vi "IterativeImputer.vi"(8 "error in":errorcluster caption="entrée d'erreur", 11 "IterativeImputer":T1={"estimator"="None", "missing_values"="nan", "sample_posterior"=FALSE, "max_iter"=10, "tol"=0.001, "n_nearest_features"=-1, "initial_strategy"="mean", "imputation_order"="ascending", "skip_complete"=FALSE, "min_value"=["None"], "max_value"=["None"], "verbose"=0, "random_state"=-1, "add_indicator"=FALSE} {"random_state" min=-1; "n_nearest_features" min=-1}) -> (0 "error out":errorcluster caption="sortie d'erreur", 3 "IterativeImputer.lvclass":refnum<class "IterativeImputer.lvclass">)   [LabVIEW 2020]
doc: "Multivariate imputer that estimates each feature from all the others.\n\nA strategy for imputing missing values by modeling each feature with missing values as a function of other features in a round-robin fashion.\n\nParameters :\n\n- estimator : object, default=BayesianRidge()\nThe estimator to use at each step of the round-robin imputation. If sample_posterior is True, the estimator must support return_std in its predict method.\n\n- missing_values : int, np.nan, default=nan\nThe placeholder for the missing values. All occurrences of missing_values will be imputed. For pandas’ dataframes with nullable integer dtypes with missing values, missing_values should be set to np.nan, since pd.NA will be converted to np.nan.\n\n- sample_posterior : boolean, default=False\nWhether to sample from the (Gaussian) predictive posterior of the fitted estimator for each imputation. Estimator must support return_std in its predict method if set to True. Set to True if using IterativeImputer for multiple imputations.\n\n- max_iter : int, default=10\nMaximum number of imputation rounds to perform before returning the imputations computed during the final round. A round is a single imputation of each feature with missing values. The stopping criterion is met once abs(max(X_t - X_{t-1}))/abs(max(X[known_vals])) < tol, where X_t is X at iteration t. Note that early stopping is only applied if ``sample_posterior=False`.\n\n- tol : float, default=1e-3\nTolerance of the stopping condition.\n\n- n_nearest_features : int, default=None=-1\nNumber of other features to use to estimate the missing values of each feature column. Nearness between features is measured using the absolute correlation coefficient between each feature pair (after initial imputation). To ensure coverage of features throughout the imputation process, the neighbor features are not necessarily nearest, but are drawn with probability proportional to correlation for each imputed target feature. Can provide significant speed-up when the number of features is huge. If None, all features will be used.\n\n- initial_strategy : str, default=’mean’\nWhich strategy to use to initialize the missing values. Same as the strategy parameter in sklearn.impute.SimpleImputer Valid values: {“mean”, “median”, “most_frequent”, or “constant”}.\n\n- imputation_order : str, default=’ascending’\nThe order in which the features will be imputed. Possible values:\n\n“ascending”\nFrom features with fewest missing values to most.\n\n“descending”\nFrom features with most missing values to fewest.\n\n“roman”\nLeft to right.\n\n“arabic”\nRight to left.\n\n“random”\nA random order for each round.\n\n- skip_complete : boolean, default=False\nIf True then features with missing values during transform which did not have any missing values during fit will be imputed with the initial imputation method only. Set to True if you have many features with no missing values at both fit and transform time to save compute.\n\n- min_value : float or array-like of shape (n_features,), default=None.\nMinimum possible imputed value. Broadcast to shape (n_features,) if scalar. If array-like, expects shape (n_features,), one min value for each feature. None (default) is converted to -np.inf.\n\n- max_value : float or array-like of shape (n_features,), default=None.\nMaximum possible imputed value. Broadcast to shape (n_features,) if scalar. If array-like, expects shape (n_features,), one max value for each feature. None (default) is converted to np.inf.\n\n- verbose : int, default=0\nVerbosity flag, controls the debug messages that are issued as functions are evaluated. The higher, the more verbose. Can be 0, 1, or 2.\n\n- random_state : int, RandomState instance or None, default=None=-1\nThe seed of the pseudo random number generator to use. Randomizes selection of estimator features if n_nearest_features is not None, the imputation_order if random, and the sampling from posterior if sample_posterior is True. Use an integer for determinism. See the Glossary.\n\n- add_indicatorboolean, default=False\nIf True, a MissingIndicator transform will stack onto output of the imputer’s transform. This allows a predictive estimator to account for missingness despite imputation. If a feature has no missing values at fit/train time, the feature won’t appear on the missing indicator even if there are missing values at transform/test time.\n\n\n\nMethods :\n\n\n- Fit : Fits the imputer on X and return self.\n\nParameters : X : array-like, shape (n_samples, n_features)\n Input data, where “n_samples” is the number of samples and “n_features” is the number of features.\n y : ignored\n\n\n- Fit Transform : Fits the imputer on X and return the transformed X.\n\nParameters : X : array-like, shape (n_samples, n_features)\n Input data, where “n_samples” is the number of samples and “n_features” is the number of features.\n y : ignored.\n\nReturns : Xt : array-like, shape (n_samples, n_features)\n The imputed input data.\n\n\n- Transform : Imputes all missing values in X.\nNote that this is stochastic, and that if random_state is not fixed, repeated calls, or permuted input, will yield different results.\n\nParameters : X : array-like of shape (n_samples, n_features)\n The input data to complete.\n\nReturns : Xt : array-like, shape (n_samples, n_features)\n The imputed input data."
uses:
  IterativeImputer.lvclass
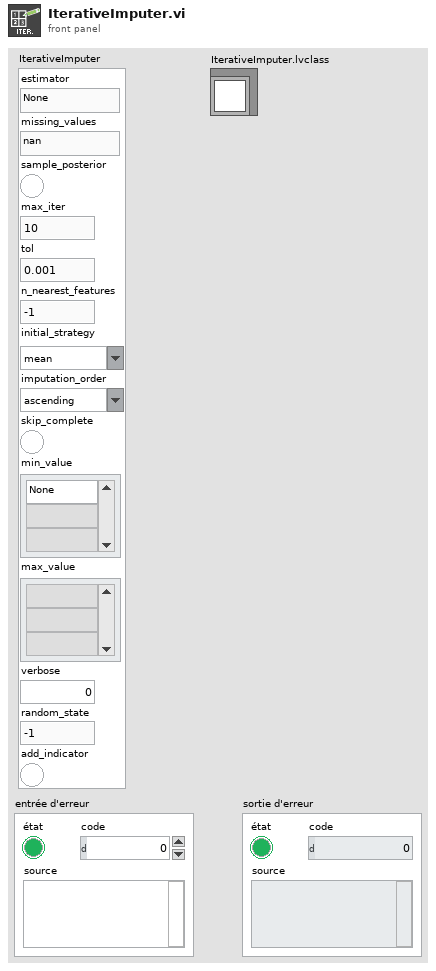
[diagram p1: front panel]
types:
  T1 = cluster{"estimator":string, "missing_values":string, "sample_posterior":bool, "max_iter":i32, "tol":dbl, "n_nearest_features":i32, "initial_strategy":string, "imputation_order":string, "skip_complete":bool, "min_value":string[], "max_value":string[], "verbose":i32, "random_state":i32, "add_indicator":bool}
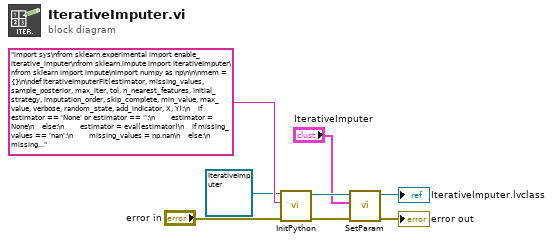
[diagram p0: block diagram]
diagram:
  n1 = call-dynamic "InitPython.vi"("error in (no error)"="error in", "Python Instruction"="import sys\nfrom sklearn.experimental import enable_iterative_imputer\nfrom sklearn.impute import IterativeImputer\nfrom sklearn import impute\nimport numpy as np\n\n\nmem = {}\n\ndef IterativeImputerFit(estimator, missing_values, sample_posterior, max_iter, tol, n_nearest_features, initial_strategy, imputation_order, skip_complete, min_value, max_value, verbose, random_state, add_indicator, X, Y):\n    if estimator == 'None' or estimator == '':\n        estimator = None\n    else:\n        estimator = eval(estimator)\n    if missing_values == 'nan':\n        missing_values = np.nan\n    else:\n        missing_values = eval(missing_values)\n    if n_nearest_features == -1:\n        n_nearest_features = None\n    if min_value == [] or min_value[0] == 'None':\n        min_value = None\n    else:\n        min_value = eval(min_value)\n    if max_value == [] or max_value[0] == 'None':\n        max_value = None\n    else:\n        max_value = eval(max_value)\n    if random_state == -1:\n        random_state = None\n    X = eval(X)\n    if Y == '':\n        Y = None\n    else:\n        Y = eval(Y)\n    try:\n        IterativeImputers = IterativeImputer(estimator, missing_values, sample_posterior, max_iter, tol, n_nearest_features, initial_strategy, imputation_order, skip_complete, min_value, max_value, verbose, random_state, add_indicator).fit(X, Y)\n        mem['FitIterativeImputer'] = IterativeImputers\n        return str('OK')\n    except:\n        erreur = sys.exc_info()\n        typerr = u\"%s\" % (erreur[0])\n        typerr = typerr[typerr.find(\"'\")+1:typerr.rfind(\"'\")]\n        msgerr = u\"%s\" % (erreur[1])\n        message = str('/!\\\\ {0} : {1}'. format(typerr,msgerr))\n        return message \n\ndef IterativeImputerFitTransform(estimator, missing_values, sample_posterior, max_iter, tol, n_nearest_features, initial_strategy, imputation_order, skip_complete, min_value, max_value, verbose, random_state, add_indicator, X, Y):\n    if estimator == 'None' or estimator == '':\n        estimator = None\n    else:\n        estimator = eval(estimator)\n    if missing_values == 'nan':\n        missing_values = np.nan\n    else:\n        missing_values = eval(missing_values)\n    if n_nearest_features == -1:\n        n_nearest_features = None\n    if min_value == [] or min_value[0] == 'None':\n        min_value = None\n    else:\n        min_value = eval(min_value)\n    if max_value == [] or max_value[0] == 'None':\n        max_value = None\n    else:\n        max_value = eval(max_value)\n    if random_state == -1:\n        random_state = None\n    X = eval(X)\n    if Y == '':\n        Y = None\n    else:\n        Y = eval(Y)\n    try:\n        IterativeImputers = IterativeImputer(estimator, missing_values, sample_posterior, max_iter, tol, n_nearest_features, initial_strategy, imputation_order, skip_complete, min_value, max_value, verbose, random_state, add_indicator).fit_transform(X, Y)\n        IterativeImputers = IterativeImputers.tolist()\n        return str(IterativeImputers)\n    except:\n        erreur = sys.exc_info()\n        typerr = u\"%s\" % (erreur[0])\n        typerr = typerr[typerr.find(\"'\")+1:typerr.rfind(\"'\")]\n        msgerr = u\"%s\" % (erreur[1])\n        message = str('/!\\\\ {0} : {1}'. format(typerr,msgerr))\n        return message \n    \n\ndef IterativeImputerTransform(estimator, missing_values, sample_posterior, max_iter, tol, n_nearest_features, initial_strategy, imputation_order, skip_complete, min_value, max_value, verbose, random_state, add_indicator, X, Y):  \n    if estimator == 'None' or estimator == '':\n        estimator = None\n    else:\n        estimator = eval(estimator)\n    if missing_values == 'nan':\n        missing_values = np.nan\n    else:\n        missing_values = eval(missing_values)\n    if n_nearest_features == -1:\n        n_nearest_features = None\n    if min_value == [] or min_value[0] == 'None':\n        min_value = None\n    else:\n        min_value = eval(min_value)\n    if max_value == [] or max_value[0] == 'None':\n        max_value = None\n    else:\n        max_value = eval(max_value)\n    if random_state == -1:\n        random_state = None\n    X = eval(X)\n    if Y == '':\n        Y = None\n    else:\n        Y = eval(Y)\n    try:\n        IterativeImputer = mem['FitIterativeImputer'].transform(X, Y)\n        IterativeImputer = IterativeImputer.tolist()\n        return str(IterativeImputer)\n    except:\n        erreur = sys.exc_info()\n        typerr = u\"%s\" % (erreur[0])\n        typerr = typerr[typerr.find(\"'\")+1:typerr.rfind(\"'\")]\n        msgerr = u\"%s\" % (erreur[1])\n        message = str('/!\\\\ {0} : {1}'. format(typerr,msgerr))\n        return message", "Scikit-learn en entrée"=refnum<class "IterativeImputer.lvclass"> refnum ("IterativeImputer.lvclass")) -> ("error out"=w6:errorcluster, "Scikit-learn en sortie"=w5:refnum<class "IterativeImputer.lvclass">)  [unwired: 7 in]
  n2 = call-dynamic "SetParam.vi"("error in (no error)"=w6, "IterativeImputer"="IterativeImputer", "IterativeImputer.lvclass"=w5) -> ("error out"=→"error out":errorcluster, "IterativeImputer.lvclass"=→"IterativeImputer.lvclass":refnum<class "IterativeImputer.lvclass">)  [unwired: 7 in]
